vi "Write Ramp Volt.vi"(8 "error in":errorcluster, 10 "Voltage_Ramp":dbl, 11 "36234A in":refnum<class "36234A.lvclass">) -> (0 "error out":errorcluster, 3 "36234A out":refnum<class "36234A.lvclass">)   [LabVIEW 2019, in "36234A.lvlib" / "36234A.lvclass"]
uses:
  Library/36234A.lvclass
  C:/Users/Public/Documents/Development/builds/Instruments/PowerSupply.lvlibp/Library/PowerSupply.lvclass
  Library/36234A.lvclass/36234A.ctl
  builds/Instruments/PowerSupply.lvlibp/Accessors/Read Active Channel.vi
  builds/Instruments/PowerSupply.lvlibp/Library/PowerSupply.lvclass
  <instrlib>/Keysight E36000 Series/Keysight E36000 Series.lvlib
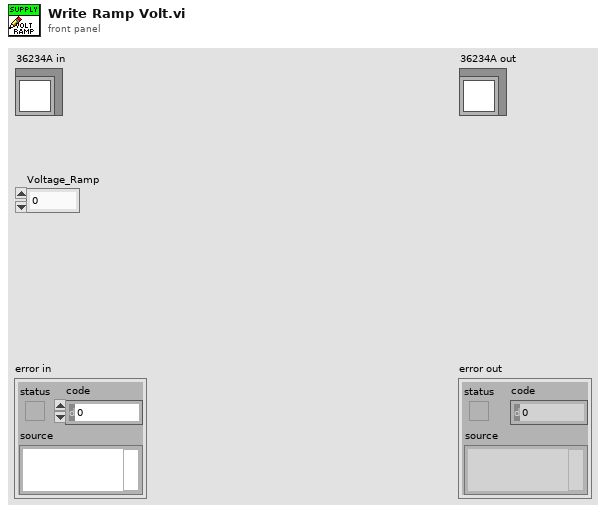
[diagram p1: front panel]
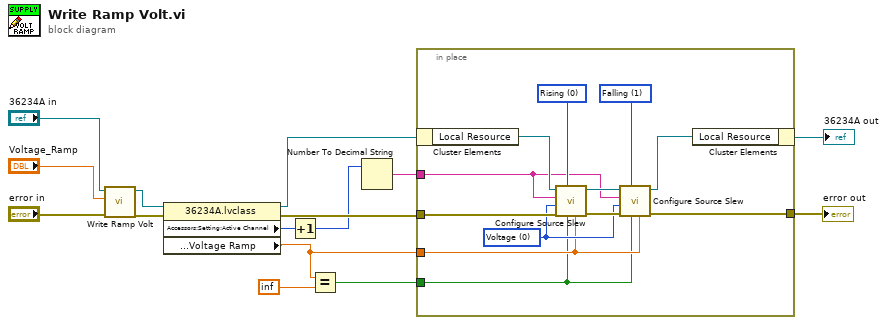
[diagram p0: block diagram]
diagram:
  n1 = call-parent "Write Ramp Volt.vi"("error in"="error in", "Voltage_Ramp"="Voltage_Ramp", "PowerSupply in"="36234A in") -> ("error out"=w8:errorcluster, "PowerSupply out"=w9:refnum<class "36234A.lvclass">)  [unwired: 7 in]
  n2 = property class="36234A.lvclass"(reference=w9, error in=w8) -> (reference out=w7:refnum<class "36234A.lvclass">, error out=w6:errorcluster, "Accessors:Setting:Active Channel"=w5:u32, "Accessors:Setting:Ramp:Voltage Ramp"=w1:dbl)
  n3 = Increment(x=w5) -> (x+1=w3:u32)
  n4 = Equal?(x=w1, y=inf) -> (x = y?=w2:bool)
  n5 = Number To Decimal String(number=w3) -> (decimal integer string=w12:string)  [unwired: 1 in]
  n6 = in-place {
    in-place-border: w6 -> [w27]
    in-place-border: [w21] -> w10
    in-place-border: w1 -> [w17]
    in-place-border: w12 -> [w18]
    in-place-border: w2 -> [w16]
    w19 = u16 1 items=["Rising", "Falling"] ("Slew Type (0: Rising)")
    w20 = u16 0 items=["Voltage", "Current", "Power", "Resistance"] ("Measurement Mode (0: Voltage)")
    w25 = u16 0 items=["Rising", "Falling"] ("Slew Type (0: Rising)")
    n7 = in-place-cluster #1(w7) -> ("Local Resource"=w26:refnum<visa-resource-name>)
    n8 = call <instrlib>:"Configure Source Slew.vi"("Slew Rate (9.9E+37)"=w17, "Enable Maximum Slew Rate (F: Disable)"=w16, "Slew Type (0: Rising)"=w25, "error in (no error)"=w27, "Measurement Mode (0: Voltage)"=w20, "Channel (1)"=w18, "VISA resource name"=w26) -> ("error out"=w24:errorcluster, "VISA resource name out"=w23:refnum<visa-resource-name>)  [unwired: 3 in]
    n9 = call <instrlib>:"Configure Source Slew.vi"("Slew Rate (9.9E+37)"=w17, "Enable Maximum Slew Rate (F: Disable)"=w16, "Slew Type (0: Rising)"=w19, "error in (no error)"=w24, "Measurement Mode (0: Voltage)"=w20, "Channel (1)"=w18, "VISA resource name"=w23) -> ("error out"=w21:errorcluster, "VISA resource name out"=w22:refnum<visa-resource-name>)  [unwired: 3 in]
    n10 = in-place-cluster #1("Local Resource"=w22) -> (→"36234A out":refnum<class "36234A.lvclass">)
  }
  "error out" <- w10
